vi "Find Neighbours 3D.vi"(10 "Position 2":T1, 11 "Position 1":T1) -> (2 "Neighbouring":bool)   [LabVIEW 2021]
uses:
  Positions 3D.ctl
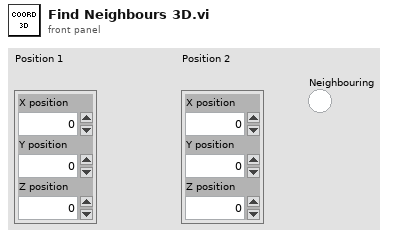
[diagram p1: front panel]
types:
  T1 = typedef "Positions 3D.ctl" = cluster{"X position":i32, "Y position":i32, "Z position":i32}
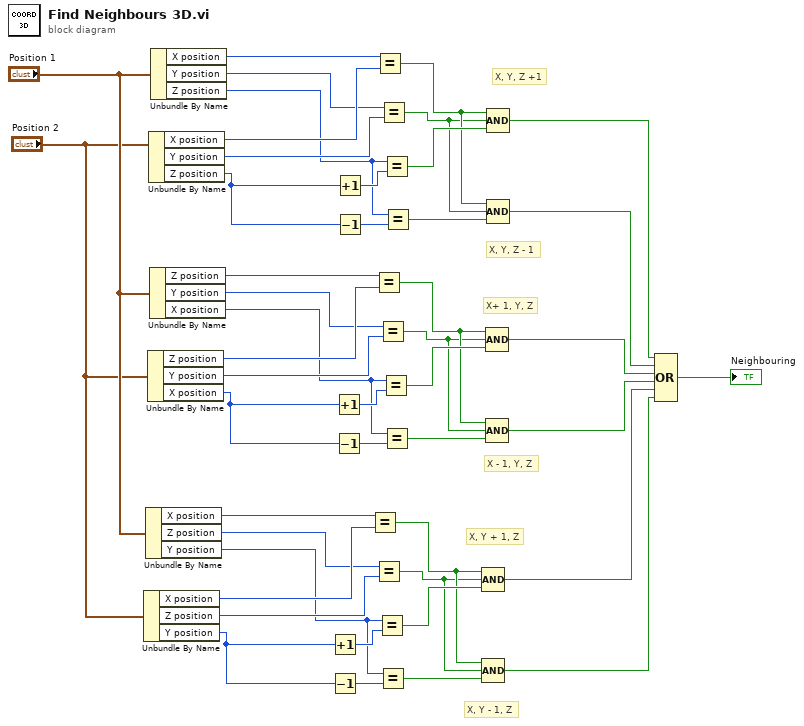
[diagram p0: block diagram]
diagram:
  # "X, Y - 1, Z"
  # "X, Y + 1, Z"
  # "X - 1, Y, Z"
  # "X+ 1, Y, Z"
  # "X, Y, Z - 1"
  # "X, Y, Z +1"
  n1 = Unbundle By Name("Position 2") -> ("X position"=w20:i32, "Z position"=w18:i32, "Y position"=w13:i32)
  n2 = Unbundle By Name("Position 1") -> ("X position"=w21:i32, "Z position"=w19:i32, "Y position"=w11:i32)
  n3 = Unbundle By Name("Position 2") -> ("Z position"=w32:i32, "Y position"=w30:i32, "X position"=w25:i32)
  n4 = Unbundle By Name("Position 2") -> ("X position"=w44:i32, "Y position"=w42:i32, "Z position"=w37:i32)
  n5 = Unbundle By Name("Position 1") -> ("Z position"=w33:i32, "Y position"=w31:i32, "X position"=w23:i32)
  n6 = Unbundle By Name("Position 1") -> ("X position"=w45:i32, "Y position"=w43:i32, "Z position"=w35:i32)
  n7 = Increment(x=w13) -> (x+1=w17:i32)
  n8 = Decrement(x=w13) -> (x-1=w12:i32)
  n9 = Increment(x=w25) -> (x+1=w29:i32)
  n10 = Decrement(x=w25) -> (x-1=w24:i32)
  n11 = Increment(x=w37) -> (x+1=w41:i32)
  n12 = Decrement(x=w37) -> (x-1=w36:i32)
  n13 = Equal?(x=w21, y=w20) -> (x = y?=w15:bool)
  n14 = Equal?(x=w33, y=w32) -> (x = y?=w27:bool)
  n15 = Equal?(x=w19, y=w18) -> (x = y?=w14:bool)
  n16 = Equal?(x=w45, y=w44) -> (x = y?=w39:bool)
  n17 = Equal?(x=w11, y=w17) -> (x = y?=w16:bool)
  n18 = Equal?(x=w31, y=w30) -> (x = y?=w26:bool)
  n19 = Equal?(x=w11, y=w12) -> (x = y?=w10:bool)
  n20 = Equal?(x=w43, y=w42) -> (x = y?=w38:bool)
  n21 = Equal?(x=w23, y=w29) -> (x = y?=w28:bool)
  n22 = Equal?(x=w35, y=w41) -> (x = y?=w40:bool)
  n23 = Equal?(x=w23, y=w24) -> (x = y?=w22:bool)
  n24 = Equal?(x=w35, y=w36) -> (x = y?=w34:bool)
  n25 = Compound Arithmetic op=AND(w15, w14, w16) -> (w3:bool)
  n26 = Compound Arithmetic op=AND(w15, w14, w10) -> (w2:bool)
  n27 = Compound Arithmetic op=AND(w27, w26, w28) -> (w5:bool)
  n28 = Compound Arithmetic op=AND(w27, w26, w22) -> (w4:bool)
  n29 = Compound Arithmetic op=AND(w39, w38, w40) -> (w7:bool)
  n30 = Compound Arithmetic op=AND(w39, w38, w34) -> (w6:bool)
  n31 = Compound Arithmetic op=OR(w7, w6, w5, w4, w3, w2) -> (→"Neighbouring":bool)
